vi "OpenStageEditorDialog.vi"(0 "System no.":i32=1 min=1 max=4 step=1, 1 "Database":enum16{"PIStages", "UserStages"}(ring), 5 "error in":errorcluster) -> (14 "DLL I32 Return value":i32, 19 "error out":errorcluster)   [LabVIEW 2020]
doc: "This VI calls the PIStageEditor which can be used to view/change stage parameters and/or add new stages. To view parameters of PI stages, select PIStages in Database. To add stages and/or change parameters, select UserStages in Database. GCSTranslator.dll and the corresponding system specific GCS DLL must be installed. The VI reads the system name from Global 2 and calls the corresponding DLL function."
uses:
  Communication/Global1.vi
  GeneralCommands/Global2 (Array).vi
panel:
  # "This vi calls the PIStageEditor which can be used to\nview/change stage parameters and/or add new stages. \nTo view parameters of PI stages, select PIStages in\n\"Database\". To add stages and/or change parameters,\nselect UserStages in \"Database\". GCSTranslator.dll and \nthe corresponding system specific GCS DLL must be \ninstalled. The VI reads the system name from Global 2 \nand calls the corresponding DLL function."
  # "General inputs:"
  # "Error handling:"
  # "DLL output:"
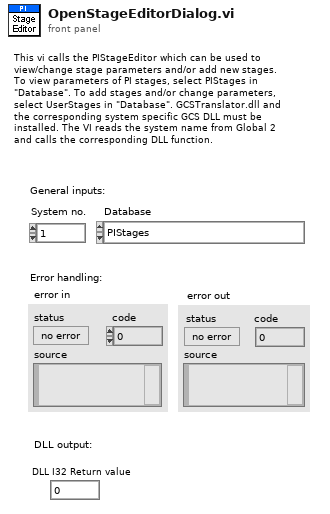
[diagram p1: front panel]
types:
  T1 = typedef "Controller names.ctl" = enum16{"None", "Analog", "C-702", "C-413", "C-414", "C-843", "C-843.PM", "C-844", "C-848", "C-865", "C-866", "C-867", "C-877", "C-880", "C-884", "C-885", "C-886", "C-887", "C-891", "E-135", "E-516", "E-517", "E-518", "E-709", "E-710", "E-712", "E-725", "E-727", "E-753", "E-754", "E-755", "E-761", "E-816", "E-861", "E-870", "E-871", "E-872", "E-873", "E-874", "F-206", "HydraPollux", "M-840", "M-850", "M-8X0", "Mercury", "Mercury_GCS", "PI_GCS2"}
  T2 = cluster{"Conn. axes":string[], "Controller name":T1}[]
  T3 = cluster{"Conn. axes":string[], "Controller name":T1}
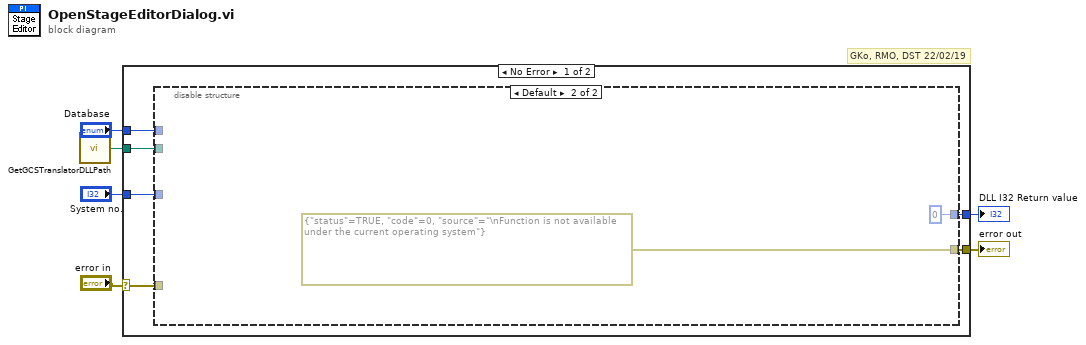
[diagram p0: block diagram]
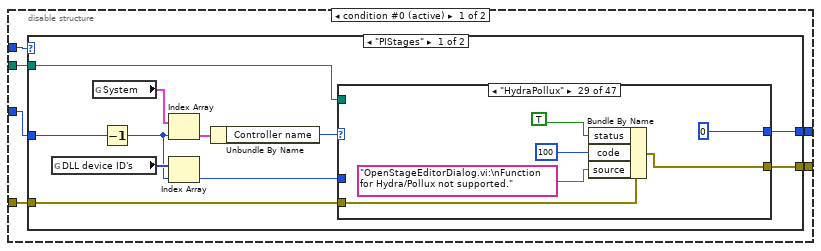
[diagram p2: hidden frame]
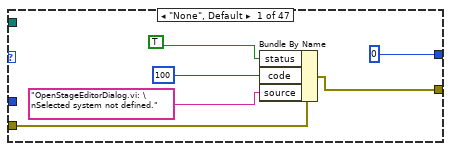
[diagram p3: hidden frame]
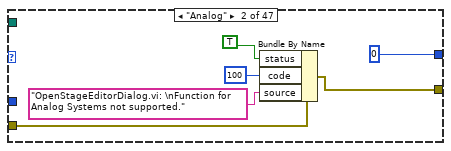
[diagram p4: hidden frame]
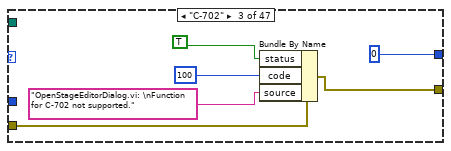
[diagram p5: hidden frame]
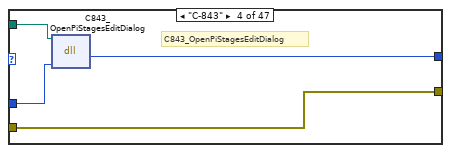
[diagram p6: hidden frame]
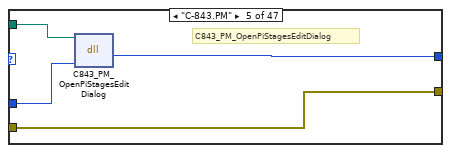
[diagram p7: hidden frame]
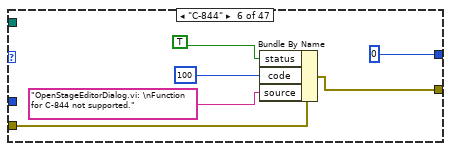
[diagram p8: hidden frame]
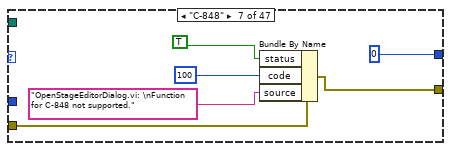
[diagram p9: hidden frame]
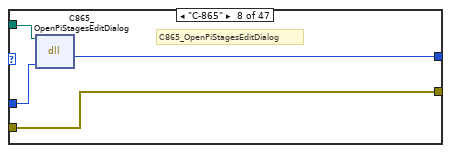
[diagram p10: hidden frame]
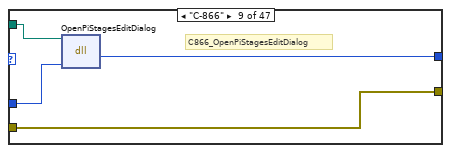
[diagram p11: hidden frame]
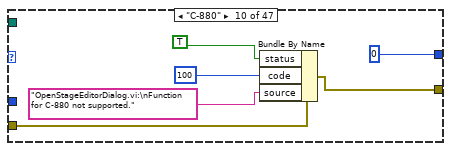
[diagram p12: hidden frame]
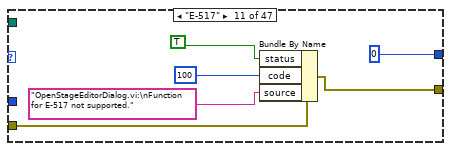
[diagram p13: hidden frame]
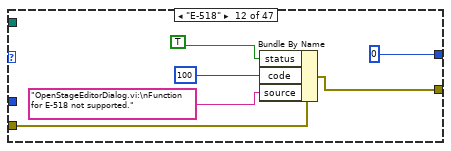
[diagram p14: hidden frame]
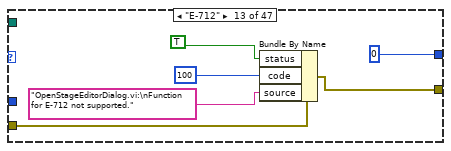
[diagram p15: hidden frame]
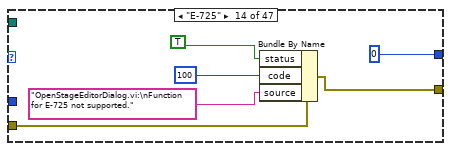
[diagram p16: hidden frame]
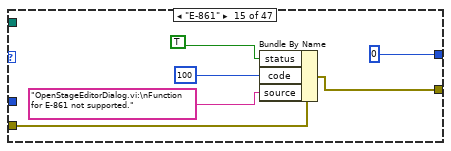
[diagram p17: hidden frame]
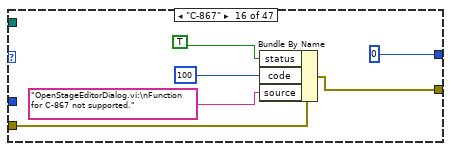
[diagram p18: hidden frame]
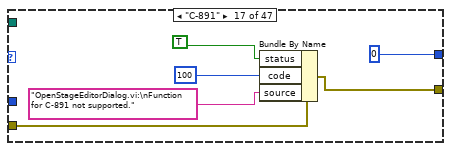
[diagram p19: hidden frame]
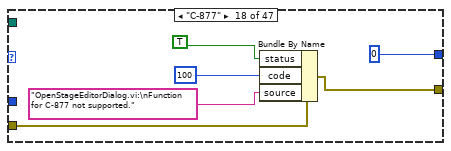
[diagram p20: hidden frame]
diagram:
  # "GKo, RMO, DST 22/02/19"
  n1 = call "GetGCSTranslatorDLLPath.vi"() -> ("DLL path"=w1:path)  [unwired: 1 in]
  n2 = case shown="No Error" "error in" {
    selector: "error in" -> [w10 w591]
    tunnel: [w12 w591] -> w6
    tunnel: [w11 0] -> w5
    tunnel: "Database" -> [w9 _]
    tunnel: "System no." -> [w8 _]
    tunnel: w1 -> [w7 _]
    frame No Error {
      n3 = disable-structure shown="Default" {
        disable-tunnel: w9 -> [w18 _]
        disable-tunnel: [w17 errorcluster {"status"=TRUE, "code"=0, "source"="\nFunction is not available under the current operating system"} ("error IO")] -> w12
        disable-tunnel: [w16 0 ("return type")] -> w11
        disable-tunnel: w8 -> [w15 _]
        disable-tunnel: w10 -> [w14 _]
        disable-tunnel: w7 -> [w13 _]
        frame condition #0 (active) {
          n4 = case shown="\"PIStages\"" w18 {
            tunnel: w15 -> [w28 w313]
            tunnel: w14 -> [w25 w310]
            tunnel: [w24 w309] -> w17
            tunnel: [w29 w314] -> w16
            tunnel: w13 -> [w19 w304]
            frame "PIStages" {
              n5 = global read "Global1.vi" "DLL device ID's"() -> (w27:i32[])
              n6 = global read "Global2 (Array).vi" "System"() -> (w22:T2)
              n7 = Decrement(x=w28) -> (x-1=w23:i32)
              n8 = Index Array(array=w22, index=w23) -> (element=w21:T3)
              n9 = Index Array(array=w27, index=w23) -> (element=w26:i32)
              n10 = Unbundle By Name(w21) -> ("Controller name"=w20:T1)
              n11 = case shown="\"HydraPollux\"" w20 {
                tunnel: [0 0 0 w51 w55 0 0 w71 w75 0 0 0 0 0 0 0 0 0 0 0 0 0 0 0 0 0 0 0 0 0 0 0 0 0 0 0 0 0 0 0 0 0 0 0 0 0 0] -> w29
                tunnel: w26 -> [_ _ _ w50 w54 _ _ w70 w74 _ _ _ _ _ _ _ _ _ _ _ _ _ _ _ _ _ _ _ _ _ _ _ _ _ _ _ _ _ _ _ _ _ _ _ _ _ _]
                tunnel: [w33 w39 w45 w49 w53 w59 w65 w69 w73 w79 w85 w91 w97 w103 w109 w115 w121 w127 w133 w139 w145 w151 w157 w163 w169 w175 w181 w187 w193 w199 w205 w211 w217 w223 w229 w235 w241 w247 w253 w259 w265 w271 w277 w283 w289 w295 w301] -> w24
                tunnel: w25 -> [w34 w40 w46 w49 w53 w60 w66 w69 w73 w80 w86 w92 w98 w104 w110 w116 w122 w128 w134 w140 w146 w152 w158 w164 w170 w176 w182 w188 w194 w200 w206 w212 w218 w224 w230 w236 w242 w248 w254 w260 w266 w272 w278 w284 w290 w296 w302]
                tunnel: w19 -> [_ _ _ w48 w52 _ _ w68 w72 _ _ _ _ _ _ _ _ _ _ _ _ _ _ _ _ _ _ _ _ _ _ _ _ _ _ _ _ _ _ _ _ _ _ _ _ _ _]
                frame "None", Default {
                  n12 = Bundle By Name(cluster=w34, "status"=TRUE, "code"=100, "source"="OpenStageEditorDialog.vi: \nSelected system not defined.") -> (w33:errorcluster)
                }
                frame "Analog" {
                  n13 = Bundle By Name(cluster=w40, "status"=TRUE, "code"=100, "source"="OpenStageEditorDialog.vi: \nFunction for Analog Systems not supported.") -> (w39:errorcluster)
                }
                frame "C-702" {
                  n14 = Bundle By Name(cluster=w46, "status"=TRUE, "code"=100, "source"="OpenStageEditorDialog.vi: \nFunction for C-702 not supported.") -> (w45:errorcluster)
                }
                frame "C-843" {
                  # "C843_OpenPiStagesEditDialog"
                  n15 = dll-call lib="T:/Entwicklung/HostSoftware/LabVIEW/GCSDrivers/source/GCS2LabVIEW/Low Level/GCSTranslator.dll" fn="C843_OpenPiStagesEditDialog"(path in=w48, "ID"=w50) -> ("return type"=w51:i32)  [unwired: 3 in, 2 out]
                }
                frame "C-843.PM" {
                  # "C843_PM_OpenPiStagesEditDialog"
                  n16 = dll-call lib="T:/Entwicklung/HostSoftware/LabVIEW/GCSDrivers/source/GCS2LabVIEW/Low Level/GCSTranslator.dll" fn="C843_PM_OpenPiStagesEditDialog"(path in=w52, "ID"=w54) -> ("return type"=w55:i32)  [unwired: 3 in, 2 out]
                }
                frame "C-844" {
                  n17 = Bundle By Name(cluster=w60, "status"=TRUE, "code"=100, "source"="OpenStageEditorDialog.vi: \nFunction for C-844 not supported.") -> (w59:errorcluster)
                }
                frame "C-848" {
                  n18 = Bundle By Name(cluster=w66, "status"=TRUE, "code"=100, "source"="OpenStageEditorDialog.vi: \nFunction for C-848 not supported.") -> (w65:errorcluster)
                }
                frame "C-865" {
                  # "C865_OpenPiStagesEditDialog"
                  n19 = dll-call lib="T:/Entwicklung/HostSoftware/LabVIEW/GCSDrivers/source/GCS2LabVIEW/Low Level/GCSTranslator.dll" fn="C865_OpenPiStagesEditDialog"(path in=w68, "ID"=w70) -> ("return type"=w71:i32)  [unwired: 3 in, 2 out]
                }
                frame "C-866" {
                  # "C866_OpenPiStagesEditDialog"
                  n20 = dll-call lib="T:/Entwicklung/HostSoftware/LabVIEW/GCSDrivers/source/GCS2LabVIEW/Low Level/GCSTranslator.dll" fn="OpenPiStagesEditDialog"(path in=w72, "ID"=w74) -> ("return type"=w75:i32)  [unwired: 3 in, 2 out]
                }
                frame "C-880" {
                  n21 = Bundle By Name(cluster=w80, "status"=TRUE, "code"=100, "source"="OpenStageEditorDialog.vi:\nFunction for C-880 not supported.") -> (w79:errorcluster)
                }
                frame "E-517" {
                  n22 = Bundle By Name(cluster=w86, "status"=TRUE, "code"=100, "source"="OpenStageEditorDialog.vi:\nFunction for E-517 not supported.") -> (w85:errorcluster)
                }
                frame "E-518" {
                  n23 = Bundle By Name(cluster=w92, "status"=TRUE, "code"=100, "source"="OpenStageEditorDialog.vi:\nFunction for E-518 not supported.") -> (w91:errorcluster)
                }
                frame "E-712" {
                  n24 = Bundle By Name(cluster=w98, "status"=TRUE, "code"=100, "source"="OpenStageEditorDialog.vi:\nFunction for E-712 not supported.") -> (w97:errorcluster)
                }
                frame "E-725" {
                  n25 = Bundle By Name(cluster=w104, "status"=TRUE, "code"=100, "source"="OpenStageEditorDialog.vi:\nFunction for E-725 not supported.") -> (w103:errorcluster)
                }
                frame "E-861" {
                  n26 = Bundle By Name(cluster=w110, "status"=TRUE, "code"=100, "source"="OpenStageEditorDialog.vi:\nFunction for E-861 not supported.") -> (w109:errorcluster)
                }
                frame "C-867" {
                  n27 = Bundle By Name(cluster=w116, "status"=TRUE, "code"=100, "source"="OpenStageEditorDialog.vi:\nFunction for C-867 not supported.") -> (w115:errorcluster)
                }
                frame "C-891" {
                  n28 = Bundle By Name(cluster=w122, "status"=TRUE, "code"=100, "source"="OpenStageEditorDialog.vi:\nFunction for C-891 not supported.") -> (w121:errorcluster)
                }
                frame "C-877" {
                  n29 = Bundle By Name(cluster=w128, "status"=TRUE, "code"=100, "source"="OpenStageEditorDialog.vi:\nFunction for C-877 not supported.") -> (w127:errorcluster)
                }
                frame "C-884" {
                  n30 = Bundle By Name(cluster=w134, "status"=TRUE, "code"=100, "source"="OpenStageEditorDialog.vi:\nFunction for C-884 not supported.") -> (w133:errorcluster)
                }
                frame "C-885" {
                  n31 = Bundle By Name(cluster=w140, "status"=TRUE, "code"=100, "source"="OpenStageEditorDialog.vi:\nFunction for C-885 not supported.") -> (w139:errorcluster)
                }
                frame "C-886" {
                  n32 = Bundle By Name(cluster=w146, "status"=TRUE, "code"=100, "source"="OpenStageEditorDialog.vi:\nFunction for C-886 not supported.") -> (w145:errorcluster)
                }
                frame "C-887" {
                  n33 = Bundle By Name(cluster=w152, "status"=TRUE, "code"=100, "source"="OpenStageEditorDialog.vi:\nFunction for C-887 not supported.") -> (w151:errorcluster)
                }
                frame "PI_GCS2" {
                  n34 = Bundle By Name(cluster=w158, "status"=TRUE, "code"=100, "source"="OpenStageEditorDialog.vi:\nFunction for PI_GCS_2 not supported.") -> (w157:errorcluster)
                }
                frame "E-709" {
                  n35 = Bundle By Name(cluster=w164, "status"=TRUE, "code"=100, "source"="OpenStageEditorDialog.vi:\nFunction for E-709 not supported.") -> (w163:errorcluster)
                }
                frame "E-870" {
                  n36 = Bundle By Name(cluster=w170, "status"=TRUE, "code"=100, "source"="OpenStageEditorDialog.vi:\nFunction for E-870 not supported.") -> (w169:errorcluster)
                }
                frame "E-871" {
                  n37 = Bundle By Name(cluster=w176, "status"=TRUE, "code"=100, "source"="OpenStageEditorDialog.vi:\nFunction for E-871 not supported.") -> (w175:errorcluster)
                }
                frame "E-872" {
                  n38 = Bundle By Name(cluster=w182, "status"=TRUE, "code"=100, "source"="OpenStageEditorDialog.vi:\nFunction for E-872 not supported.") -> (w181:errorcluster)
                }
                frame "E-874" {
                  n39 = Bundle By Name(cluster=w188, "status"=TRUE, "code"=100, "source"="OpenStageEditorDialog.vi:\nFunction for E-874 not supported.") -> (w187:errorcluster)
                }
                frame "HydraPollux" {
                  n40 = Bundle By Name(cluster=w194, "status"=TRUE, "code"=100, "source"="OpenStageEditorDialog.vi:\nFunction for Hydra/Pollux not supported.") -> (w193:errorcluster)
                }
                frame "Mercury_GCS" {
                  n41 = Bundle By Name(cluster=w200, "status"=TRUE, "code"=100, "source"="OpenStageEditorDialog.vi:\nFunction for Mercury_GCS not supported.") -> (w199:errorcluster)
                }
                frame "C-413" {
                  n42 = Bundle By Name(cluster=w206, "status"=TRUE, "code"=100, "source"="OpenStageEditorDialog.vi:\nFunction for C-413 not supported.") -> (w205:errorcluster)
                }
                frame "C-414" {
                  n43 = Bundle By Name(cluster=w212, "status"=TRUE, "code"=100, "source"="OpenStageEditorDialog.vi:\nFunction for C-414 not supported.") -> (w211:errorcluster)
                }
                frame "E-516" {
                  n44 = Bundle By Name(cluster=w218, "status"=TRUE, "code"=100, "source"="OpenStageEditorDialog.vi: \nFunction for E-516 not supported.") -> (w217:errorcluster)
                }
                frame "E-710" {
                  n45 = Bundle By Name(cluster=w224, "status"=TRUE, "code"=100, "source"="OpenStageEditorDialog.vi: \nFunction for E-710 not supported.") -> (w223:errorcluster)
                }
                frame "E-753" {
                  n46 = Bundle By Name(cluster=w230, "status"=TRUE, "code"=100, "source"="OpenStageEditorDialog.vi: \nFunction for E-753 not supported.") -> (w229:errorcluster)
                }
                frame "E-727" {
                  n47 = Bundle By Name(cluster=w236, "status"=TRUE, "code"=100, "source"="OpenStageEditorDialog.vi: \nFunction for E-727 not supported.") -> (w235:errorcluster)
                }
                frame "E-873" {
                  n48 = Bundle By Name(cluster=w242, "status"=TRUE, "code"=100, "source"="OpenStageEditorDialog.vi: \nFunction for E-873 not supported.") -> (w241:errorcluster)
                }
                frame "E-754" {
                  n49 = Bundle By Name(cluster=w248, "status"=TRUE, "code"=100, "source"="OpenStageEditorDialog.vi: \nFunction for E-754 not supported.") -> (w247:errorcluster)
                }
                frame "E-755" {
                  n50 = Bundle By Name(cluster=w254, "status"=TRUE, "code"=100, "source"="OpenStageEditorDialog.vi: \nFunction for E-755 not supported.") -> (w253:errorcluster)
                }
                frame "E-761" {
                  n51 = Bundle By Name(cluster=w260, "status"=TRUE, "code"=100, "source"="OpenStageEditorDialog.vi: \nFunction for E-761 not supported.") -> (w259:errorcluster)
                }
                frame "E-816" {
                  n52 = Bundle By Name(cluster=w266, "status"=TRUE, "code"=100, "source"="OpenStageEditorDialog.vi: \nFunction for E-816 not supported.") -> (w265:errorcluster)
                }
                frame "F-206" {
                  n53 = Bundle By Name(cluster=w272, "status"=TRUE, "code"=100, "source"="OpenStageEditorDialog.vi: \nFunction for F-206 not supported.") -> (w271:errorcluster)
                }
                frame "M-840" {
                  n54 = Bundle By Name(cluster=w278, "status"=TRUE, "code"=100, "source"="OpenStageEditorDialog.vi: \nFunction for M-840 not supported.") -> (w277:errorcluster)
                }
                frame "E-135" {
                  n55 = Bundle By Name(cluster=w284, "status"=TRUE, "code"=100, "source"="OpenStageEditorDialog.vi: \nFunction for E-135 not supported.") -> (w283:errorcluster)
                }
                frame "M-850" {
                  n56 = Bundle By Name(cluster=w290, "status"=TRUE, "code"=100, "source"="OpenStageEditorDialog.vi: \nFunction for M-850 not supported.") -> (w289:errorcluster)
                }
                frame "M-8X0" {
                  n57 = Bundle By Name(cluster=w296, "status"=TRUE, "code"=100, "source"="OpenStageEditorDialog.vi: \nFunction for M-8X0 not supported.") -> (w295:errorcluster)
                }
                frame "Mercury" {
                  n58 = Bundle By Name(cluster=w302, "status"=TRUE, "code"=100, "source"="OpenStageEditorDialog.vi: \nFunction for Mercury not supported.") -> (w301:errorcluster)
                }
              }
            }
            frame "UserStages" {
              n59 = global read "Global1.vi" "DLL device ID's"() -> (w312:i32[])
              n60 = global read "Global2 (Array).vi" "System"() -> (w306:T2)
              n61 = Decrement(x=w313) -> (x-1=w307:i32)
              n62 = Index Array(array=w306, index=w307) -> (element=w308:T3)
              n63 = Index Array(array=w312, index=w307) -> (element=w311:i32)
              n64 = Unbundle By Name(w308) -> ("Controller name"=w305:T1)
              n65 = case shown="\"C-413\"" w305 {
                tunnel: [0 0 0 w336 w340 0 0 w356 w360 0 0 0 0 0 0 0 0 0 0 0 0 0 0 0 0 0 0 0 0 0 0 0 0 0 0 0 0 0 0 0 0 0 0 0 0 0 0] -> w314
                tunnel: w311 -> [_ _ _ w335 w339 _ _ w355 w359 _ _ _ _ _ _ _ _ _ _ _ _ _ _ _ _ _ _ _ _ _ _ _ _ _ _ _ _ _ _ _ _ _ _ _ _ _ _]
                tunnel: w310 -> [w316 w322 w328 w334 w338 w342 w348 w354 w358 w362 w368 w374 w380 w386 w392 w398 w404 w410 w416 w422 w428 w434 w440 w446 w452 w458 w464 w470 w476 w482 w488 w494 w500 w506 w512 w518 w524 w530 w536 w542 w548 w554 w560 w566 w572 w578 w584]
                tunnel: [w315 w321 w327 w334 w338 w341 w347 w354 w358 w361 w367 w373 w379 w385 w391 w397 w403 w409 w415 w421 w427 w433 w439 w445 w451 w457 w463 w469 w475 w481 w487 w493 w499 w505 w511 w517 w523 w529 w535 w541 w547 w553 w559 w565 w571 w577 w583] -> w309
                tunnel: w304 -> [_ _ _ w333 w337 _ _ w353 w357 _ _ _ _ _ _ _ _ _ _ _ _ _ _ _ _ _ _ _ _ _ _ _ _ _ _ _ _ _ _ _ _ _ _ _ _ _ _]
                frame "None", Default {
                  n66 = Bundle By Name(cluster=w316, "status"=TRUE, "code"=100, "source"="OpenStageEditorDialog.vi: \nSelected system not defined.") -> (w315:errorcluster)
                }
                frame "Analog" {
                  n67 = Bundle By Name(cluster=w322, "status"=TRUE, "code"=100, "source"="OpenStageEditorDialog.vi: \nFunction for Analog systems not supported.") -> (w321:errorcluster)
                }
                frame "C-702" {
                  n68 = Bundle By Name(cluster=w328, "status"=TRUE, "code"=100, "source"="OpenStageEditorDialog.vi: \nFunction for C-702 not supported.") -> (w327:errorcluster)
                }
                frame "C-843" {
                  # "C843_OpenUserStagesEditDialog"
                  n69 = dll-call lib="T:/Entwicklung/HostSoftware/LabVIEW/GCSDrivers/source/GCS2LabVIEW/Low Level/GCSTranslator.dll" fn="C843_OpenUserStagesEditDialog"(path in=w333, "ID"=w335) -> ("return type"=w336:i32)  [unwired: 3 in, 2 out]
                }
                frame "C-843.PM" {
                  # "C843_PM_OpenUserStagesEditDialog"
                  n70 = dll-call lib="T:/Entwicklung/HostSoftware/LabVIEW/GCSDrivers/source/GCS2LabVIEW/Low Level/GCSTranslator.dll" fn="C843_PM_OpenUserStagesEditDialog"(path in=w337, "ID"=w339) -> ("return type"=w340:i32)  [unwired: 3 in, 2 out]
                }
                frame "C-844" {
                  n71 = Bundle By Name(cluster=w342, "status"=TRUE, "code"=100, "source"="OpenStageEditorDialog.vi: \nFunction for C-844 not supported.") -> (w341:errorcluster)
                }
                frame "C-848" {
                  n72 = Bundle By Name(cluster=w348, "status"=TRUE, "code"=100, "source"="OpenStageEditorDialog.vi: \nFunction for C-848 not supported.") -> (w347:errorcluster)
                }
                frame "C-865" {
                  # "C865_OpenUserStagesEditDialog"
                  n73 = dll-call lib="T:/Entwicklung/HostSoftware/LabVIEW/GCSDrivers/source/GCS2LabVIEW/Low Level/GCSTranslator.dll" fn="C865_OpenUserStagesEditDialog"(path in=w353, "ID"=w355) -> ("return type"=w356:i32)  [unwired: 3 in, 2 out]
                }
                frame "C-866" {
                  # "C866_OpenUserStagesEditDialog"
                  n74 = dll-call lib="T:/Entwicklung/HostSoftware/LabVIEW/GCSDrivers/source/GCS2LabVIEW/Low Level/GCSTranslator.dll" fn="OpenUserStagesEditDialog"(path in=w357, "ID"=w359) -> ("return type"=w360:i32)  [unwired: 3 in, 2 out]
                }
                frame "C-880" {
                  n75 = Bundle By Name(cluster=w362, "status"=TRUE, "code"=100, "source"="OpenStageEditorDialog.vi: \nFunction for C-880 not supported.") -> (w361:errorcluster)
                }
                frame "E-517" {
                  n76 = Bundle By Name(cluster=w368, "status"=TRUE, "code"=100, "source"="OpenStageEditorDialog.vi: \nFunction for E-517 not supported.") -> (w367:errorcluster)
                }
                frame "E-518" {
                  n77 = Bundle By Name(cluster=w374, "status"=TRUE, "code"=100, "source"="OpenStageEditorDialog.vi: \nFunction for E-518 not supported.") -> (w373:errorcluster)
                }
                frame "E-712" {
                  n78 = Bundle By Name(cluster=w380, "status"=TRUE, "code"=100, "source"="OpenStageEditorDialog.vi: \nFunction for E-712 not supported.") -> (w379:errorcluster)
                }
                frame "E-725" {
                  n79 = Bundle By Name(cluster=w386, "status"=TRUE, "code"=100, "source"="OpenStageEditorDialog.vi: \nFunction for E-725 not supported.") -> (w385:errorcluster)
                }
                frame "E-861" {
                  n80 = Bundle By Name(cluster=w392, "status"=TRUE, "code"=100, "source"="OpenStageEditorDialog.vi: \nFunction for E-861 not supported.") -> (w391:errorcluster)
                }
                frame "C-867" {
                  n81 = Bundle By Name(cluster=w398, "status"=TRUE, "code"=100, "source"="OpenStageEditorDialog.vi: \nFunction for C-867 not supported.") -> (w397:errorcluster)
                }
                frame "C-891" {
                  n82 = Bundle By Name(cluster=w404, "status"=TRUE, "code"=100, "source"="OpenStageEditorDialog.vi: \nFunction for C-891 not supported.") -> (w403:errorcluster)
                }
                frame "C-877" {
                  n83 = Bundle By Name(cluster=w410, "status"=TRUE, "code"=100, "source"="OpenStageEditorDialog.vi: \nFunction for C-877 not supported.") -> (w409:errorcluster)
                }
                frame "E-516" {
                  n84 = Bundle By Name(cluster=w416, "status"=TRUE, "code"=100, "source"="OpenStageEditorDialog.vi: \nFunction for E-516 not supported.") -> (w415:errorcluster)
                }
                frame "E-710" {
                  n85 = Bundle By Name(cluster=w422, "status"=TRUE, "code"=100, "source"="OpenStageEditorDialog.vi: \nFunction for E-710 not supported.") -> (w421:errorcluster)
                }
                frame "E-753" {
                  n86 = Bundle By Name(cluster=w428, "status"=TRUE, "code"=100, "source"="OpenStageEditorDialog.vi: \nFunction for E-753 not supported.") -> (w427:errorcluster)
                }
                frame "HydraPollux" {
                  n87 = Bundle By Name(cluster=w434, "status"=TRUE, "code"=100, "source"="OpenStageEditorDialog.vi: \nFunction for Hydra/Pollux not supported.") -> (w433:errorcluster)
                }
                frame "Mercury_GCS" {
                  n88 = Bundle By Name(cluster=w440, "status"=TRUE, "code"=100, "source"="OpenStageEditorDialog.vi: \nFunction for Mercury_GCS not supported.") -> (w439:errorcluster)
                }
                frame "C-413" {
                  n89 = Bundle By Name(cluster=w446, "status"=TRUE, "code"=100, "source"="OpenStageEditorDialog.vi: \nFunction for C-413 not supported.") -> (w445:errorcluster)
                }
                frame "C-414" {
                  n90 = Bundle By Name(cluster=w452, "status"=TRUE, "code"=100, "source"="OpenStageEditorDialog.vi: \nFunction for C-414 not supported.") -> (w451:errorcluster)
                }
                frame "E-135" {
                  n91 = Bundle By Name(cluster=w458, "status"=TRUE, "code"=100, "source"="OpenStageEditorDialog.vi: \nFunction for E-135 not supported.") -> (w457:errorcluster)
                }
                frame "PI_GCS2" {
                  n92 = Bundle By Name(cluster=w464, "status"=TRUE, "code"=100, "source"="OpenStageEditorDialog.vi: \nFunction for PI_GCS_2 not supported.") -> (w463:errorcluster)
                }
                frame "C-884" {
                  n93 = Bundle By Name(cluster=w470, "status"=TRUE, "code"=100, "source"="OpenStageEditorDialog.vi: \nFunction for C-884 not supported.") -> (w469:errorcluster)
                }
                frame "C-885" {
                  n94 = Bundle By Name(cluster=w476, "status"=TRUE, "code"=100, "source"="OpenStageEditorDialog.vi: \nFunction for C-885 not supported.") -> (w475:errorcluster)
                }
                frame "C-886" {
                  n95 = Bundle By Name(cluster=w482, "status"=TRUE, "code"=100, "source"="OpenStageEditorDialog.vi: \nFunction for C-886 not supported.") -> (w481:errorcluster)
                }
                frame "C-887" {
                  n96 = Bundle By Name(cluster=w488, "status"=TRUE, "code"=100, "source"="OpenStageEditorDialog.vi: \nFunction for C-887 not supported.") -> (w487:errorcluster)
                }
                frame "E-709" {
                  n97 = Bundle By Name(cluster=w494, "status"=TRUE, "code"=100, "source"="OpenStageEditorDialog.vi: \nFunction for E-709 not supported.") -> (w493:errorcluster)
                }
                frame "E-727" {
                  n98 = Bundle By Name(cluster=w500, "status"=TRUE, "code"=100, "source"="OpenStageEditorDialog.vi: \nFunction for E-727 not supported.") -> (w499:errorcluster)
                }
                frame "E-870" {
                  n99 = Bundle By Name(cluster=w506, "status"=TRUE, "code"=100, "source"="OpenStageEditorDialog.vi: \nFunction for E-870 not supported.") -> (w505:errorcluster)
                }
                frame "E-871" {
                  n100 = Bundle By Name(cluster=w512, "status"=TRUE, "code"=100, "source"="OpenStageEditorDialog.vi: \nFunction for E-871 not supported.") -> (w511:errorcluster)
                }
                frame "E-872" {
                  n101 = Bundle By Name(cluster=w518, "status"=TRUE, "code"=100, "source"="OpenStageEditorDialog.vi: \nFunction for E-872 not supported.") -> (w517:errorcluster)
                }
                frame "E-873" {
                  n102 = Bundle By Name(cluster=w524, "status"=TRUE, "code"=100, "source"="OpenStageEditorDialog.vi: \nFunction for E-873 not supported.") -> (w523:errorcluster)
                }
                frame "E-874" {
                  n103 = Bundle By Name(cluster=w530, "status"=TRUE, "code"=100, "source"="OpenStageEditorDialog.vi: \nFunction for E-874 not supported.") -> (w529:errorcluster)
                }
                frame "E-754" {
                  n104 = Bundle By Name(cluster=w536, "status"=TRUE, "code"=100, "source"="OpenStageEditorDialog.vi: \nFunction for E-754 not supported.") -> (w535:errorcluster)
                }
                frame "E-755" {
                  n105 = Bundle By Name(cluster=w542, "status"=TRUE, "code"=100, "source"="OpenStageEditorDialog.vi: \nFunction for E-755 not supported.") -> (w541:errorcluster)
                }
                frame "E-761" {
                  n106 = Bundle By Name(cluster=w548, "status"=TRUE, "code"=100, "source"="OpenStageEditorDialog.vi: \nFunction for E-761 not supported.") -> (w547:errorcluster)
                }
                frame "E-816" {
                  n107 = Bundle By Name(cluster=w554, "status"=TRUE, "code"=100, "source"="OpenStageEditorDialog.vi: \nFunction for E-816 not supported.") -> (w553:errorcluster)
                }
                frame "F-206" {
                  n108 = Bundle By Name(cluster=w560, "status"=TRUE, "code"=100, "source"="OpenStageEditorDialog.vi: \nFunction for F-206 not supported.") -> (w559:errorcluster)
                }
                frame "M-840" {
                  n109 = Bundle By Name(cluster=w566, "status"=TRUE, "code"=100, "source"="OpenStageEditorDialog.vi: \nFunction for M-840 not supported.") -> (w565:errorcluster)
                }
                frame "M-850" {
                  n110 = Bundle By Name(cluster=w572, "status"=TRUE, "code"=100, "source"="OpenStageEditorDialog.vi: \nFunction for M-850 not supported.") -> (w571:errorcluster)
                }
                frame "M-8X0" {
                  n111 = Bundle By Name(cluster=w578, "status"=TRUE, "code"=100, "source"="OpenStageEditorDialog.vi: \nFunction for M-8X0 not supported.") -> (w577:errorcluster)
                }
                frame "Mercury" {
                  n112 = Bundle By Name(cluster=w584, "status"=TRUE, "code"=100, "source"="OpenStageEditorDialog.vi: \nFunction for Mercury not supported.") -> (w583:errorcluster)
                }
              }
            }
          }
        }
        frame condition #1 {
        }
      }
    }
    frame Error {
    }
  }
  "error out" <- w6
  "DLL I32 Return value" <- w5
